vi "Disabled.vi"(7 "Robot Mode":T2, 10 "Match Info":T1={"Autonomous Elapsed Seconds"=0.0, "TeleOp Elapsed Seconds"=0.0, "Disabled Elapsed Seconds"=0.0, "Visited Autonomous"=FALSE, "Visited TeleOp"=FALSE, "Visited Disabled"=FALSE, "Autonomous Settings"={"Autonomous Style"=enum."Independent", "VI Refnum"=refnum}}, 11 "Call Context":T3) -> ()   [LabVIEW 2011]
doc: "This VI is called each time a disabled packet is received from the DS. It is often used to prepare for the next robot mode, to calibrate sensors, etc."
uses:
  <vilib>/Rock Robotics/WPI/DriverStation/WPI_DriverStationDerivedRobotMode.ctl
  <vilib>/Rock Robotics/WPI/DriverStation/WPI_DriverStationRobotMode.ctl
  <vilib>/Rock Robotics/WPI/DriverStation/WPI_DriverStationMatch Info.ctl
  <vilib>/Rock Robotics/WPI/Relay/WPI_RelayValue.ctl
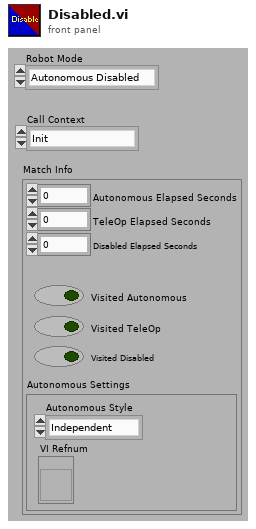
[diagram p1: front panel]
types:
  T1 = typedef "WPI_DriverStationMatch Info.ctl" = cluster{"Autonomous Elapsed Seconds":dbl, "TeleOp Elapsed Seconds":dbl, "Disabled Elapsed Seconds":dbl, "Visited Autonomous":bool, "Visited TeleOp":bool, "Visited Disabled":bool, "Autonomous Settings":cluster{"Autonomous Style":enum16{"Iterative", "Independent"}, "VI Refnum":refnum<vi>}}
  T2 = typedef "WPI_DriverStationRobotMode.ctl" = enum16{"Autonomous Disabled", "Autonomous Enabled", "Teleop Disabled", "Teleop Enabled", "Timeout", "Finish"}
  T3 = typedef "WPI_DriverStationDerivedRobotMode.ctl" = enum16{"Init", "Execute", "Stop"}
  T4 = typedef "WPI_RelayValue.ctl" = enum16{"Off", "On", "Forward", "Reverse"}
  T5 = typedef "WPI_RobotDriveDevRef.ctl" = cluster{"DevStatus":errorcluster, "Motors[]":T6[], "Square Inputs":bool, "Max Output":dbl, "Isochronous":bool}
  T6 = typedef "WPI_MotorControlDeviceRef.ctl" = cluster{"DeviceStatus":errorcluster, "Type":enum16{"PWM", "CAN"}, "PWM":cluster{"Digital Module":T7, "PWM Channel":T8, "DeadBand":T9}, "CAN":cluster{"Device Number":u8, "Control Mode":T10, "Semaphore":T11, "Max Vout":dbl}, "Invert":bool, "TransformRef":T12, "InvTransformRef":T12}
  T7 = typedef "FPGA_TypedefDigitalModule.ctl" = enum16{"Digital Module 1", "Digital Module 2"}
  T8 = typedef "FPGA_DIOPWMChannel.ctl" = enum8{"PWM 1", "PWM 2", "PWM 3", "PWM 4", "PWM 5", "PWM 6", "PWM 7", "PWM 8", "PWM 9", "PWM 10", "Invalid"}
  T9 = typedef "WPI_PWMDeadband.ctl" = cluster{"Name":string, "maxPositivePwm":i32, "minPositivePwm":i32, "centerPwm":i32, "maxNegativePwm":i32, "minNegativePwm":i32, "angularRange":u16}
  T10 = typedef "WPI_CANJaguar_ControlMode.ctl" = enum8{"Percent VBus", "Current", "Speed", "Position", "Voltage"}
  T11 = typedef "Semaphore RefNum" = refnum<k1>
  T12 = typedef "WPI_PWMTransform_ConPane.ctl" = refnum<vi>
  T13 = typedef "WPI_RelayDevRef.ctl" = cluster{"DevStatus":errorcluster, "Relay Channel":T14, "Digital Module":T7, "Relay Direction":T15}
  T14 = typedef "FPGA_DIORelayChannel.ctl" = enum8{"Relay 1", "Relay 2", "Relay 3", "Relay 4", "Relay 5", "Relay 6", "Relay 7", "Relay 8", "Invalid"}
  T15 = typedef "WPI_RelayDirection.ctl" = enum16{"Both directions", "Forward only", "Reverse only"}
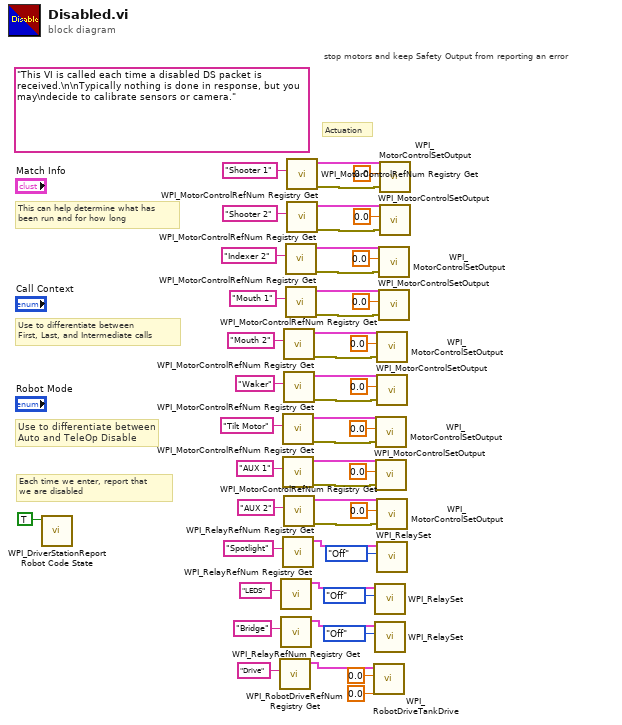
[diagram p0: block diagram]
diagram:
  (unwired) "This VI is called each time a disabled DS packet is received.\n\nTypically nothing is done in response, but you may\ndecide to calibrate sensors or camera."
  # "Actuation"
  # "Each time we enter, report that\nwe are disabled"
  # "stop motors and keep Safety Output from reporting an error"
  # "Use to differentiate between\nFirst, Last, and Intermediate calls"
  # "This can help determine what has\nbeen run and for how long"
  # "Use to differentiate between\nAuto and TeleOp Disable"
  n1 = call <vilib>:"WPI_DriverStationReport Robot Code State.vi"("Disabled"=TRUE ("Autonomous")) -> ()  [unwired: 10 in, 1 out]
  n2 = call <vilib>:"WPI_RobotDriveRefNum Registry Get.vi"("refnum name"="Drive") -> ("RobotDriveDevRef"=w3:T5)  [unwired: 9 in, 1 out]
  n3 = call <vilib>:"WPI_RelayRefNum Registry Get.vi"("refnum name"="LEDS") -> ("RelayDevRef"=w9:T13)  [unwired: 9 in, 1 out]
  n4 = call <vilib>:"WPI_RelayRefNum Registry Get.vi"("refnum name"="Bridge") -> ("RelayDevRef"=w6:T13)  [unwired: 9 in, 1 out]
  n5 = call <vilib>:"WPI_MotorControlRefNum Registry Get.vi"("refnum name"="Tilt Motor") -> ("error out"=w28:errorcluster, "MotorControlDevRef"=w25:T6)  [unwired: 9 in]
  n6 = call <vilib>:"WPI_MotorControlRefNum Registry Get.vi"("refnum name"="AUX 1") -> ("error out"=w29:errorcluster, "MotorControlDevRef"=w22:T6)  [unwired: 9 in]
  n7 = call <vilib>:"WPI_RelayRefNum Registry Get.vi"("refnum name"="Spotlight") -> ("RelayDevRef"=w12:T13)  [unwired: 9 in, 1 out]
  n8 = call <vilib>:"WPI_MotorControlRefNum Registry Get.vi"("refnum name"="Mouth 2") -> ("error out"=w26:errorcluster, "MotorControlDevRef"=w18:T6)  [unwired: 9 in]
  n9 = call <vilib>:"WPI_MotorControlRefNum Registry Get.vi"("refnum name"="Waker") -> ("error out"=w27:errorcluster, "MotorControlDevRef"=w21:T6)  [unwired: 9 in]
  n10 = call <vilib>:"WPI_MotorControlRefNum Registry Get.vi"("refnum name"="AUX 2") -> ("error out"=w15:errorcluster, "MotorControlDevRef"=w17:T6)  [unwired: 9 in]
  n11 = call <vilib>:"WPI_MotorControlRefNum Registry Get.vi"("refnum name"="Indexer 2") -> ("error out"=w39:errorcluster, "MotorControlDevRef"=w42:T6)  [unwired: 9 in]
  n12 = call <vilib>:"WPI_MotorControlRefNum Registry Get.vi"("refnum name"="Mouth 1") -> ("error out"=w38:errorcluster, "MotorControlDevRef"=w45:T6)  [unwired: 9 in]
  n13 = call <vilib>:"WPI_MotorControlRefNum Registry Get.vi"("refnum name"="Shooter 1") -> ("error out"=w41:errorcluster, "MotorControlDevRef"=w49:T6)  [unwired: 9 in]
  n14 = call <vilib>:"WPI_MotorControlRefNum Registry Get.vi"("refnum name"="Shooter 2") -> ("error out"=w40:errorcluster, "MotorControlDevRef"=w46:T6)  [unwired: 9 in]
  n15 = call <vilib>:"WPI_RobotDriveTankDrive.vi"("Right axis value"=0.0, "Left axis value"=0.0, "RobotDriveDevRef"=w3) -> ()  [unwired: 7 in, 2 out]
  n16 = call <vilib>:"WPI_RelaySet.vi"("RelayValue"=WPI_RelayValue."Off", "RelayDevRef"=w9) -> ()  [unwired: 8 in, 2 out]
  n17 = call <vilib>:"WPI_RelaySet.vi"("RelayValue"=WPI_RelayValue."Off", "RelayDevRef"=w6) -> ()  [unwired: 8 in, 2 out]
  n18 = call <vilib>:"WPI_MotorControlSetOutput.vi"("error in (no error)"=w28, "Output"=0.0, "MotorControlDevRef"=w25) -> ()  [unwired: 7 in, 2 out]
  n19 = call <vilib>:"WPI_MotorControlSetOutput.vi"("error in (no error)"=w29, "Output"=0.0, "MotorControlDevRef"=w22) -> ()  [unwired: 7 in, 2 out]
  n20 = call <vilib>:"WPI_MotorControlSetOutput.vi"("error in (no error)"=w26, "Output"=0.0, "MotorControlDevRef"=w18) -> ()  [unwired: 7 in, 2 out]
  n21 = call <vilib>:"WPI_MotorControlSetOutput.vi"("error in (no error)"=w27, "Output"=0.0, "MotorControlDevRef"=w21) -> ()  [unwired: 7 in, 2 out]
  n22 = call <vilib>:"WPI_MotorControlSetOutput.vi"("error in (no error)"=w15, "Output"=0.0, "MotorControlDevRef"=w17) -> ()  [unwired: 7 in, 2 out]
  n23 = call <vilib>:"WPI_RelaySet.vi"("RelayValue"=WPI_RelayValue."Off", "RelayDevRef"=w12) -> ()  [unwired: 8 in, 2 out]
  n24 = call <vilib>:"WPI_MotorControlSetOutput.vi"("error in (no error)"=w39, "Output"=0.0, "MotorControlDevRef"=w42) -> ()  [unwired: 7 in, 2 out]
  n25 = call <vilib>:"WPI_MotorControlSetOutput.vi"("error in (no error)"=w38, "Output"=0.0, "MotorControlDevRef"=w45) -> ()  [unwired: 7 in, 2 out]
  n26 = call <vilib>:"WPI_MotorControlSetOutput.vi"("error in (no error)"=w41, "Output"=0.0, "MotorControlDevRef"=w49) -> ()  [unwired: 7 in, 2 out]
  n27 = call <vilib>:"WPI_MotorControlSetOutput.vi"("error in (no error)"=w40, "Output"=0.0, "MotorControlDevRef"=w46) -> ()  [unwired: 7 in, 2 out]
